vi "SECoP_dataGetScale.vi"(7 "Position":u32, 8 "error in (no error)":errorcluster, 10 "SECoP_dataPtr":T1 {"ptr64" format="%.0x"; "ptr32" format="%.0x"}, 11 "DLL path (in)":T2) -> (0 "error out":errorcluster, 2 "scale factor":dbl, 3 "DLL path (out)":T2)   [LabVIEW 2023, in "SECoP.lvlib"]
doc: "Call <b>\"SECoP_dataGetScale.vi\"</b> to access the scale factor (SECoP_dataPtr).\n\n<b>DLL path</b> input and output of cluster from \"SECoP-Initialize.vi\"\n<b>SECoP_dataPtr</b> data to access\n<b>Position</b> points to a virtual flattened entry of the data type\n<b>scale factor</b> scale factor of scaled value"
uses:
  SECoP.lvlib
  SECoP-libraries.ctl
  SECoP-data.ctl
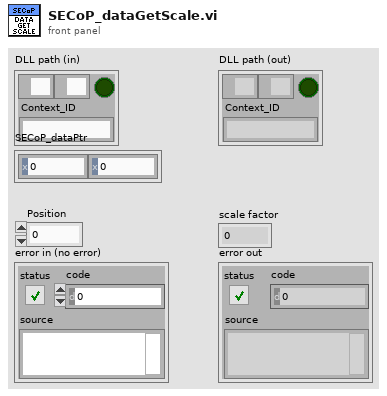
[diagram p1: front panel]
types:
  T1 = typedef "SECoP.lvlib/SECoP-data.ctl" = cluster{"ptr32":u32, "ptr64":u64}
  T2 = typedef "SECoP.lvlib/SECoP-libraries.ctl" = cluster{"serverDLL":path, "variantDLL":path, "cleanup_mode":bool, "Context_ID":string}
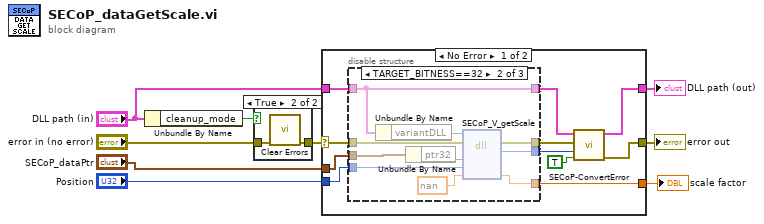
[diagram p0: block diagram]
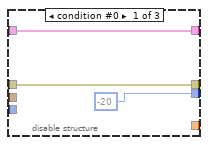
[diagram p3: hidden frame]
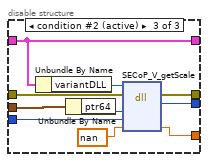
[diagram p4: hidden frame]
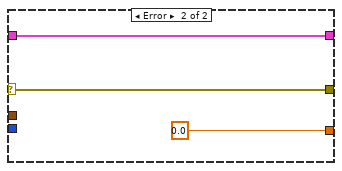
[diagram p5: hidden frame]
diagram:
  n1 = Unbundle By Name("DLL path (in)") -> ("cleanup_mode"=w6:bool)
  n2 = case shown="True" w6 {
    tunnel: "error in (no error)" -> [w10 w12]
    tunnel: [w10 w11] -> w4
    frame False {
    }
    frame True {
      n3 = call <vilib>:"Clear Errors.vi"("error in (no error)"=w12) -> ("error out"=w11:errorcluster)  [unwired: 5 in, 1 out]
    }
  }
  n4 = case shown="No Error" w4 {
    selector: w4 -> [w21 w48]
    tunnel: "DLL path (in)" -> [w20 w49]
    tunnel: [w22 w49] -> w8
    tunnel: [w23 w48] -> w7
    tunnel: "Position" -> [w15 _]
    tunnel: [w14 0.0 ("Value")] -> w2
    tunnel: "SECoP_dataPtr" -> [w13 _]
    frame No Error {
      n5 = disable-structure shown="TARGET_BITNESS==32" {
        disable-tunnel: w21 -> [w24 w36 w46]
        disable-tunnel: w20 -> [w25 w28 w37]
        disable-tunnel: [w25 w28 w37] -> w19
        disable-tunnel: [w24 w35 w45] -> w18
        disable-tunnel: [-20 w34 w44] -> w17
        disable-tunnel: w15 -> [_ w33 w43]
        disable-tunnel: [_ w32 w42] -> w14
        disable-tunnel: w13 -> [_ w30 w40]
        frame condition #0 {
        }
        frame condition #1 {
          n6 = Unbundle By Name(w28) -> ("variantDLL"=w27:path)
          n7 = Unbundle By Name(w30) -> ("ptr32"=w31:u32)
          n8 = dll-call lib="Z:/Praktische_Aufgaben/SECoP-LabVIEW2015/32bit/SECoP32.dll" fn="SECoP_V_getScale"(path in=w27, error in=w36, "pData"=w31, "uPosition"=w33, "dScale"=nan) -> (error out=w35:errorcluster, "return type"=w34:i32, "dScale"=w32:dbl)  [unwired: 3 in, 1 out]
        }
        frame condition #2 (active) {
          n9 = Unbundle By Name(w37) -> ("variantDLL"=w38:path)
          n10 = Unbundle By Name(w40) -> ("ptr64"=w41:u64)
          n11 = dll-call lib="Z:/Praktische_Aufgaben/SECoP-LabVIEW2015/32bit/SECoP32.dll" fn="SECoP_V_getScale"(path in=w38, error in=w46, "pData"=w41, "uPosition"=w43, "dScale"=nan) -> (error out=w45:errorcluster, "return type"=w44:i32, "dScale"=w42:dbl)  [unwired: 3 in, 1 out]
        }
      }
      n12 = call "SECoP-ConvertError.vi"("return is boolean"=TRUE, "return code"=w17, "error in (no error)"=w18, "DLL path (in)"=w19) -> ("error out"=w23:errorcluster, "DLL path (out)"=w22:T2)  [unwired: 6 in]
    }
    frame Error {
    }
  }
  "DLL path (out)" <- w8
  "error out" <- w7
  "scale factor" <- w2
